vi "Get Default Log File Directory.vi"(8 "error in":errorcluster, 11 "Device Item Ref In":T1 format="%.0x") -> (0 "error out":errorcluster, 2 "Log File Directory String Array":string[](array[string]), 3 "Device Item Ref Out":T1 format="%.0x")   [LabVIEW 2019, in "Telemetry System Explorer.lvlib"]
uses:
  Telemetry System Explorer.lvlib
  <vilib>/NI VeriStand/Custom Device API/Custom Device Item Ref.ctl
  <vilib>/NI VeriStand/Custom Device API/Custom Device API.lvlib
  <vilib>/NI VeriStand/Custom Device Tools/Custom Device Utility Library/Custom Device Utility Library.lvlib
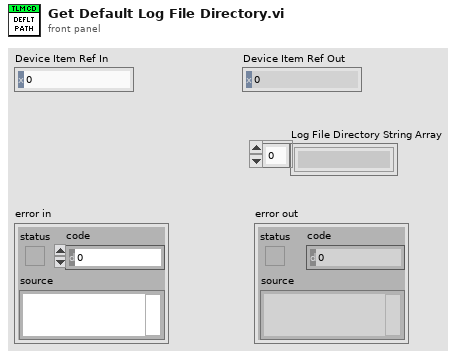
[diagram p1: front panel]
types:
  T1 = typedef "Custom Device API.lvlib/Custom Device Item Ref.ctl" = u64
  T2 = typedef "Custom Device API.lvlib/Custom Device Target Type.ctl" = enum16{"PharLap", "VxWorks", "Windows", "Linux_32_ARM", "Linux_x64"}
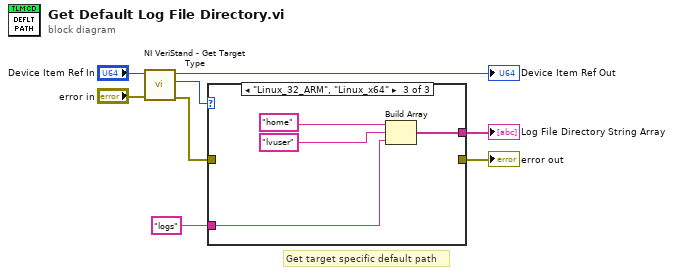
[diagram p0: block diagram]
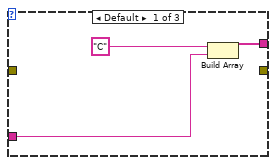
[diagram p2: hidden frame]
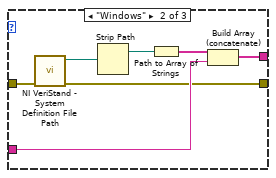
[diagram p3: hidden frame]
diagram:
  # "Get target specific default path"
  n1 = call <vilib>:"NI VeriStand - Get Target Type.vi"("error in (no error)"="error in", "Item Ref in"="Device Item Ref In") -> ("error out"=w2:errorcluster, "Target Type"=w6:T2, "Item Ref out"=→"Device Item Ref Out":T1)  [unwired: 7 in]
  n2 = case shown="\"Linux_32_ARM\", \"Linux_x64\"" w6 {
    tunnel: [w9 w17 w19] -> w8
    tunnel: "logs" -> [w10 w18 w20]
    tunnel: w2 -> [_ w16 _]
    tunnel: [_ w15 _] -> w1
    frame Default {
      n3 = Build Array("C", w10) -> (w9:string[])
    }
    frame "Windows" {
      n4 = call <vilib>:"NI VeriStand - System Definition File Path.vi"("error in (no error)"=w16) -> ("error out"=w15:errorcluster, "SDF path"=w14:path)  [unwired: 9 in]
      n5 = Strip Path(path=w14) -> (stripped path=w13:path)  [unwired: 1 out]
      n6 = Path to Array of Strings(0:w13) -> (2:w12:string[])  [unwired: 1 out]
      n7 = Build Array (concatenate)(w12, w18) -> (w17:string[])
    }
    frame "Linux_32_ARM", "Linux_x64" {
      n8 = Build Array("home", "lvuser", w20) -> (w19:string[])
    }
  }
  "Log File Directory String Array" <- w8
  "error out" <- w1
